vi "VISA resource XBee.vi"() -> ()   [LabVIEW 2017]
panel:
  in  "VISA resource name":refnum<visa-resource-name>
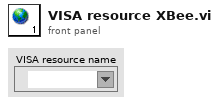
[diagram p1: front panel]
diagram:
